vi "Airportsecondstillarive.vi"() -> ()   [LabVIEW 2014]
panel:
  out "seconds(whole)":dbl
  out "min":dbl
  out "hours":dbl
  in  "seconds":dbl
  # "controll"
  # "indicator"
  # "indicator"
  # "indicator"
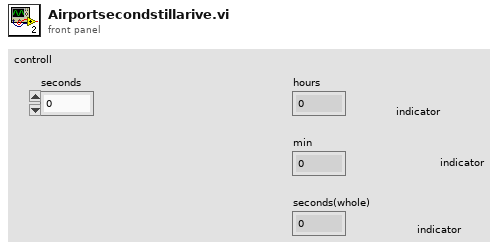
[diagram p1: front panel]
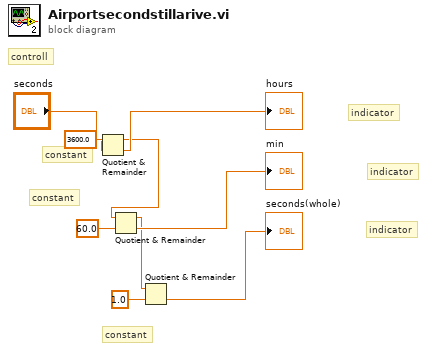
[diagram p0: block diagram]
diagram:
  # "controll"
  # "constant"
  # "constant"
  # "constant"
  # "indicator"
  # "indicator"
  # "indicator"
  n1 = Quotient & Remainder(x="seconds", y=3600.0 ("x-y*floor(x/y)")) -> (x-y*floor(x/y)=w6:dbl, floor(x/y)=→"hours":dbl)
  n2 = Quotient & Remainder(x=w6, y=60.0) -> (x-y*floor(x/y)=w3:dbl, floor(x/y)=→"min":dbl)
  n3 = Quotient & Remainder(x=w3, y=1.0) -> (floor(x/y)=→"seconds(whole)":dbl)  [unwired: 1 out]
